vi "Get Control References.vi"(7 "appended array":string[](array[string]), 8 "error in (no error)":errorcluster, 11 "Control References":refnum<vi>[](array[refnum])) -> (0 "error out":errorcluster, 2 "Control Class ID":u32[](array[numeric]), 3 "Label Name":string[][](array[string]))   [LabVIEW 2018]
uses:
  <vilib>/Math Plots/3D Math Plots/3D Surface/3D Surface XCtrl/3D Surface.xctl
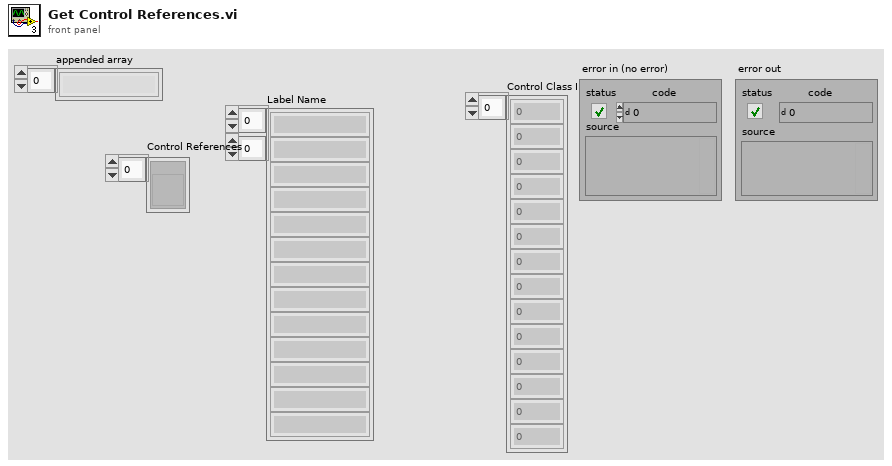
[diagram p1: front panel]
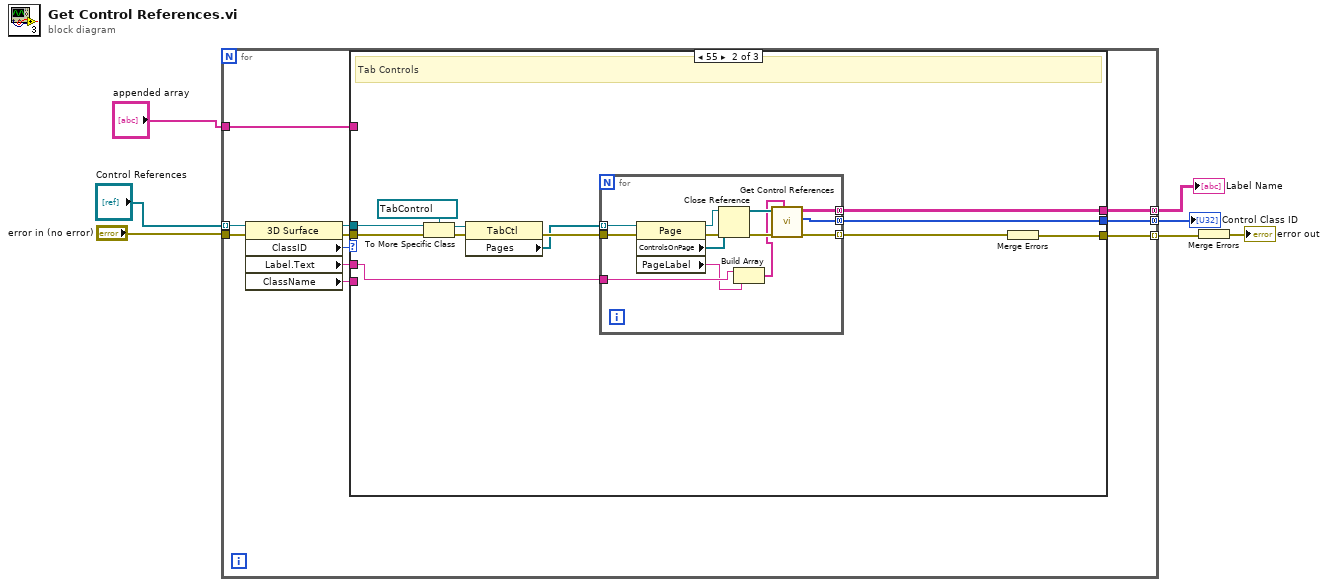
[diagram p0: block diagram]
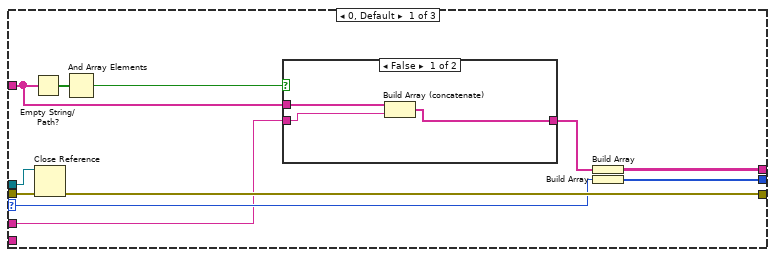
[diagram p2: hidden frame]
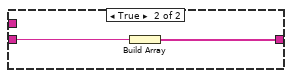
[diagram p3: hidden frame]
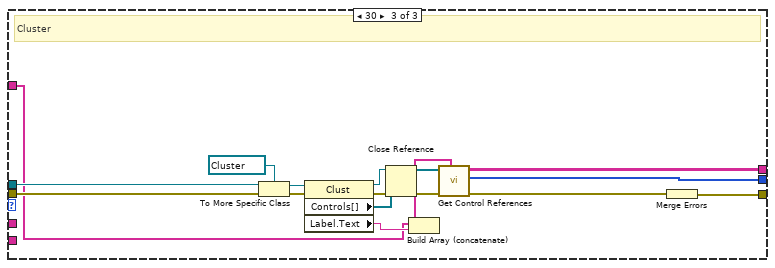
[diagram p4: hidden frame]
diagram:
  n1 = for {
    tunnel: "error in (no error)" -> [w18]
    tunnel: "Control References" -> [w13] mode=indexing
    tunnel: [w12] -> w4 mode=indexing
    tunnel: [w11] -> w2 mode=concatenating
    tunnel: [w10] -> w3 mode=concatenating
    tunnel: "appended array" -> [w8]
    n2 = property class="3D Surface"(reference=w13, error in=w18) -> (reference out=w15:refnum<vi>, error out=w14:errorcluster, "ClassID"=w17:u32, "Label.Text"=w16:string, "ClassName"=w9:string)
    n3 = case shown="55" w17 {
      selector: w17 -> [w25 _ _]
      tunnel: w16 -> [w22 w35 _]
      tunnel: w15 -> [w28 w44 w72]
      tunnel: w14 -> [w29 w46 w74]
      tunnel: [w27 w38 w69] -> w12
      tunnel: [w26 w37 w68] -> w11
      tunnel: [w19 w36 w67] -> w10
      tunnel: w9 -> [_ _ _]
      tunnel: w8 -> [w23 _ w59]
      frame 0, Default {
        n4 = Empty String/Path?(string/path=w23) -> (empty?=w24:bool[])
        n5 = Close Reference(reference=w28, error in (no error)=w29) -> (error out=w27:errorcluster)
        n6 = And Array Elements(Boolean array=w24) -> (logical AND=w20:bool)
        n7 = case shown="False" w20 {
          tunnel: w22 -> [w31 w34]
          tunnel: [w30 w33] -> w21
          tunnel: w23 -> [w32 _]
          frame False {
            n8 = Build Array (concatenate)(w32, w31) -> (w30:string[])
          }
          frame True {
            n9 = Build Array(w34) -> (w33:string[])
          }
        }
        n10 = Build Array(w21) -> (w19:string[][])
        n11 = Build Array(w25) -> (w26:u32[])
      }
      frame 55 {
        # "Tab Controls"
        n12 = To More Specific Class(target class=refnum<vi> refnum ("Control Panel"), reference=w44, error in=w46) -> (specific class reference=w43:refnum<vi>, error out=w45:errorcluster)
        n13 = property class="TabCtl"(reference=w43, error in=w45) -> (error out=w41:errorcluster, "Pages"=w40:refnum<vi>[])  [unwired: 1 out]
        n14 = for {
          tunnel: w41 -> [w58]
          tunnel: w40 -> [w56] mode=indexing
          tunnel: [w52] -> w36 mode=concatenating
          tunnel: [w51] -> w37 mode=concatenating
          tunnel: [w50] -> w39 mode=indexing
          tunnel: w35 -> [w49]
          n15 = property class="Page"(reference=w56, error in=w58) -> (reference out=w53:refnum<vi>, error out=w57:errorcluster, "ControlsOnPage"=w55:refnum<vi>[], "PageLabel"=w48:string)
          n16 = Close Reference(reference=w53, error in (no error)=w57) -> (error out=w54:errorcluster)
          n17 = Build Array(w49, w48) -> (w47:string[])
          n18 = call "Get Control References.vi"("appended array"=w47, "error in (no error)"=w54, "Control References"=w55) -> ("error out"=w50:errorcluster, "Control Class ID"=w51:u32[], "Label Name"=w52:string[][])  [unwired: 6 in]
        }
        n19 = Merge Errors(w39) -> (w38:errorcluster)
      }
      frame 30 {
        # "Cluster"
        n20 = To More Specific Class(target class=refnum<vi> refnum ("System Parameters"), reference=w72, error in=w74) -> (specific class reference=w71:refnum<vi>, error out=w73:errorcluster)
        n21 = property class="Clust"(reference=w71, error in=w73) -> (reference out=w62:refnum<vi>, error out=w64:errorcluster, "Controls[]"=w63:refnum<vi>[], "Label.Text"=w60:string)
        n22 = Close Reference(reference=w62, error in (no error)=w64) -> (error out=w65:errorcluster)
        n23 = Build Array (concatenate)(w59, w60) -> (w61:string[])
        n24 = call "Get Control References.vi"("appended array"=w61, "error in (no error)"=w65, "Control References"=w63) -> ("error out"=w70:errorcluster, "Control Class ID"=w68:u32[], "Label Name"=w67:string[][])  [unwired: 6 in]
        n25 = Merge Errors(w70) -> (w69:errorcluster)
      }
    }
  }
  "Label Name" <- w3
  "Control Class ID" <- w2
  n26 = Merge Errors(w4) -> (→"error out":errorcluster)
